vi "get_uvars.vi"(0 "SEQs in":T1[](array[typedef])) -> (2 "SEQs out":T1[](array[typedef]), 3 "UVARS":string[](array[string]), 4 "vVARS":variant)   [LabVIEW 2013]
uses:
  Line.ctl
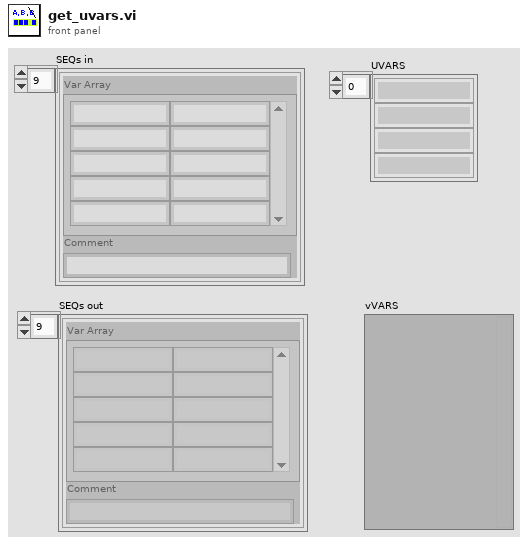
[diagram p1: front panel]
types:
  T1 = typedef "Line.ctl" = cluster{"Var Array":string[][], "Comment":string}
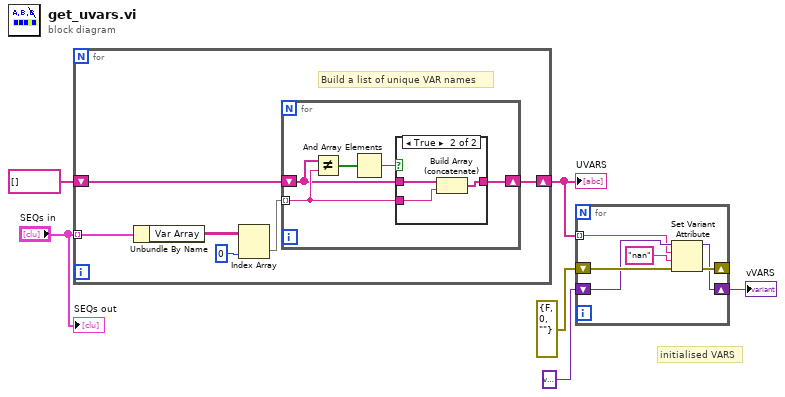
[diagram p0: block diagram]
diagram:
  # "initialised VARS"
  n1 = for {
    tunnel: "SEQs in" -> [w12] mode=indexing
    shift-right: [w7] -> w3
    shift-left: string[] [] -> [w10]
    # "Build a list of unique VAR names"
    n2 = Unbundle By Name(w12) -> ("Var Array"=w11:string[][])
    n3 = Index Array(array=w11, index (col)=0 ("disabled index (col)")) -> (element=w8:string[])  [unwired: 1 in]
    n4 = for {
      tunnel: w8 -> [w17] mode=indexing
      shift-right: [w15] -> w7
      shift-left: w10 -> [w16]
      n5 = Not Equal?(x=w16, y=w17) -> (x != y?=w14:bool[])
      n6 = And Array Elements(Boolean array=w14) -> (logical AND=w13:bool)
      n7 = case shown="True" w13 {
        tunnel: w17 -> [_ w21]
        tunnel: w16 -> [w18 w20]
        tunnel: [w18 w19] -> w15
        frame False {
        }
        frame True {
          n8 = Build Array (concatenate)(w20, w21) -> (w19:string[])
        }
      }
    }
  }
  "UVARS" <- w3
  n9 = for {
    shift-right: [w24] -> w1
    shift-left: variant ("duplicate variant") -> [w25]
    tunnel: w3 -> [w23] mode=indexing
    shift-right: [w26] -> _
    shift-left: errorcluster {"status"=FALSE, "code"=0, "source"=""} ("error in") -> [w27]
    n10 = Set Variant Attribute(Variant=w25, name=w23, value="nan", error in=w27) -> (Variant out=w24:variant, error out=w26:errorcluster)  [unwired: 1 out]
  }
  "vVARS" <- w1
  "SEQs out" <- "SEQs in"
